vi "Uniform (Discrete) Moments.vi"(10 "n":i32=100) -> (0 "error":i32, 2 "variance":dbl=833.25, 3 "mean":dbl=50.5)   [LabVIEW 2020, in "NI_Gmath.lvlib"]
doc: "Returns the expected mean and variance of the random variate X, where X describes the selected distribution type. You must manually select the polymorphic instance to use."
uses:
  NI_Gmath.lvlib
  st_error_code.ctl
panel:
  # "Uniform (Discrete) Moments"
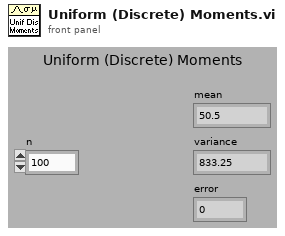
[diagram p1: front panel]
types:
  T1 = typedef "NI_Gmath.lvlib/st_error_code.ctl" = i32
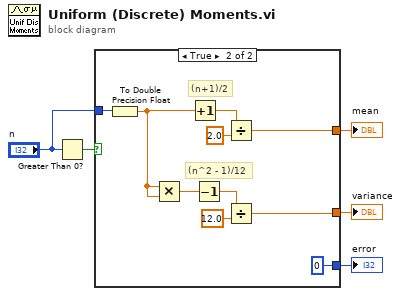
[diagram p0: block diagram]
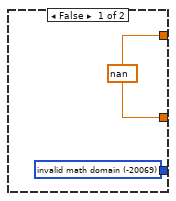
[diagram p2: hidden frame]
diagram:
  n1 = Greater Than 0?(x="n") -> (x > 0?=w5:bool)
  n2 = case shown="True" w5 {
    tunnel: [w6 0 ("invalid math domain")] -> w4
    tunnel: [w7 w15] -> w3
    tunnel: [w7 w10] -> w2
    tunnel: "n" -> [_ w14]
    frame False {
      w6 = T1 -20069 items=["invalid math domain"=-20069, "Fourier interpolation size m >= n"=-20070, "empty array"=-20003] ("stat interp error code")
      w7 = nan
    }
    frame True {
      # "(n^2 - 1)/12"
      # "(n+1)/2"
      n3 = To Double Precision Float(number=w14) -> (double precision float=w9:dbl)
      n4 = Multiply(x=w9, y=w9) -> (x*y=w13:dbl)
      n5 = Increment(x=w9) -> (x+1=w16:dbl)
      n6 = Decrement(x=w13) -> (x-1=w11:dbl)
      n7 = Divide(x=w16, y=2.0) -> (x/y=w15:dbl)
      n8 = Divide(x=w11, y=12.0) -> (x/y=w10:dbl)
    }
  }
  "mean" <- w3
  "error" <- w4
  "variance" <- w2
